vi "Configure Thermocouple [TC].vi"(8 "error in (no error)":errorcluster, 9 "ref junc type (Internal)":i32(ring)=1 items=["Internal"=1, "Fixed"=2], 10 "thermocouple type (B)":i32(ring)=1 items=["B"=1, "C"=2, "D"=3, "E"=4, "G"=5, "J"=6, "K"=7, "N"=8, "R"=9, "S"=10, "T"=11, "U"=12, "V"=13], 11 "CS++DMM in":refnum<class "CS++DMM.lvclass">) -> (0 "error out":errorcluster, 3 "CS++DMM out":refnum<class "CS++DMM.lvclass">)   [LabVIEW 2016, in "CS++DMM.lvlib" / "CS++DMM.lvclass"]
doc: "This VI configures the thermocouple type and the reference junction type of the thermocouple for DMMs that take temperature measurements using a thermocouple transducer type.\n\nThis VI affects the behavior of the instrument only if the IviDmm>Temperature Measurements>Transducer Type [TMP] property is set to IVIDMM_VAL_THERMOCOUPLE. \n\nNote:\n\n(1) This VI is part of the IviDmmThermocouple [TC] extension group."
uses:
  CS++DMM.lvclass
  CSPP_Core/Classes/CS++ProcessVariables/ProcessVariable/PV.lvclass
  PV-Enum.ctl
  CS++DMM.lvclass/CS++DMM.ctl
  CSPP_Core/Classes/CS++ProcessVariables/ProcessVariable/PV.lvclass/PV.ctl
  CSPP_Core/Classes/CS++ProcessVariables/ProcessVariable/Write Data.vi
  CSPP_Core/Classes/CS++ProcessVariables/ProcessVariable/Write Timestamp.vi
  CSPP_Core/Classes/CS++ProcessVariables/ProcessVariable/Write Quality.vi
  CSPP_Core/Classes/CS++ProcessVariables/ProcessVariable/Write status.vi
  CSPP_Core/Classes/CS++ProcessVariables/PVConnection/PVConnection.lvclass
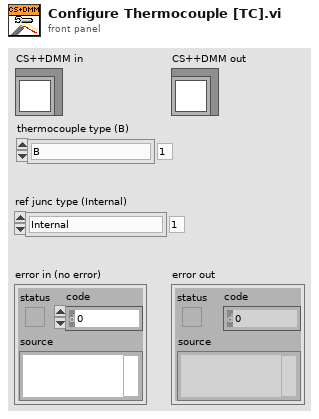
[diagram p1: front panel]
types:
  T1 = typedef "CS++DMM.lvlib/CS++DMM.lvclass/PV-Enum.ctl" = enum16{"AbsoluteResolution", "ACMaxFrequency", "ACMinFrequency", "ActualRange", "Alpha", "ApertureTime", "FixedReferenceJunction", "FrequencyVoltageRange", "PowerLineFrequency", "Range", "Reading", "Resistance", "SampleInterval", "TriggerDelay", "ApertureTimeUnit", "AutoZeroMode", "MeasCompleteDestination", "MeasurementFunction", "ReferenceJunctionType", "SampleCount", "SampleTrigger", "ThermocoupleType", "TransducerType", "TriggerCount", "TriggerSlope", "TriggerSource", "MPReading", "IsOverRange"}
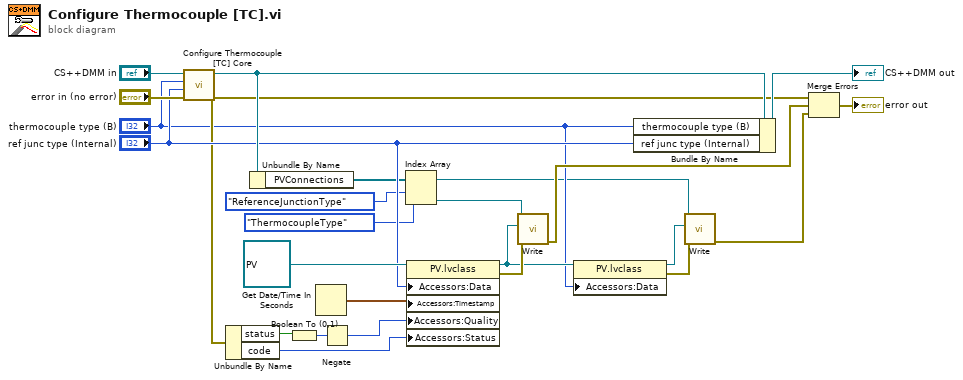
[diagram p0: block diagram]
diagram:
  n1 = call-dynamic "Configure Thermocouple [TC] Core.vi"("error in (no error)"="error in (no error)", "ref junc type (Internal)"="ref junc type (Internal)", "thermocouple type (B)"="thermocouple type (B)", "CS++DMM in"="CS++DMM in") -> ("error out"=w11:errorcluster, "CS++DMM out"=w15:refnum<class "CS++DMM.lvclass">)  [unwired: 6 in]
  n2 = Unbundle By Name(w11) -> ("status"=w21:bool, "code"=w18:i32)
  n3 = Unbundle By Name(w15) -> ("PVConnections"=w6:refnum<class "PVConnection.lvclass">[])
  n4 = Boolean To (0,1)(Boolean=w21) -> (0, 1=w20:i16)
  n5 = Get Date/Time In Seconds() -> (seconds since 1Jan1904=w17:timestamp)
  n6 = Negate(x=w20) -> (-x=w19:i16)
  n7 = Index Array(array=w6, index #1=PV-Enum."ReferenceJunctionType" ("PV-Enum"), index #2=PV-Enum."ThermocoupleType" ("PV-Enum")) -> (element #1=w4:refnum<class "PVConnection.lvclass">, element #2=w1:refnum<class "PVConnection.lvclass">)
  n8 = property class="PV.lvclass"(reference=refnum<class "PV.lvclass"> refnum ("CS++ProcessVariables.lvlib:PV.lvclass"), "Accessors:Data"="ref junc type (Internal)", "Accessors:Timestamp"=w17, "Accessors:Quality"=w19, "Accessors:Status"=w18) -> (reference out=w9:refnum<class "PV.lvclass">, error out=w16:errorcluster)  [unwired: 1 in]
  n9 = call "Write.vi"("error in (no error)"=w16, "PV"=w9, "PVConnection in"=w1) -> ("error out"=w10:errorcluster)  [unwired: 7 in, 1 out]
  n10 = property class="PV.lvclass"(reference=w9, "Accessors:Data"="thermocouple type (B)") -> (reference out=w12:refnum<class "PV.lvclass">, error out=w13:errorcluster)  [unwired: 1 in]
  n11 = Bundle By Name(cluster=w15, "thermocouple type (B)"="thermocouple type (B)", "ref junc type (Internal)"="ref junc type (Internal)") -> (→"CS++DMM out":refnum<class "CS++DMM.lvclass">)
  n12 = call "Write.vi"("error in (no error)"=w13, "PV"=w12, "PVConnection in"=w4) -> ("error out"=w7:errorcluster)  [unwired: 7 in, 1 out]
  n13 = Merge Errors(w11, w10, w7) -> (→"error out":errorcluster)
